vi "test_serialize_deserialize.vi"   [LabVIEW 2020, in "Waveform(DBL) Array.lvlib"]
doc: "Version 0.1"
uses:
  <vilib>/ADAS Record/CustomDataTypes/Waveform(DBL) Array/Waveform(DBL) Array.lvlib
  <vilib>/addons/_JKI Toolkits/Caraya/classes/Test/Test.lvclass
  <vilib>/addons/_JKI Toolkits/Caraya/classes/Assert/Assert.lvclass
  <vilib>/ADAS Record/CustomDataTypes/Waveform(DBL) Array/Process Data.ctl
  <vilib>/ADAS Record/CustomDataTypes/ADAS Generic/Serialize Data.vi
  <vilib>/ADAS Record/CustomDataTypes/ADAS Generic/NI_ADAS_Generic.lvlib
  <vilib>/ADAS Record/CustomDataTypes/ADAS Generic/Deserialize Data.vi
types:
  T1 = typedef "Waveform(DBL) Array.lvlib/Process Data.ctl" = cluster{"Waveform(dbl) Array":waveform(dbl)[]}
  T2 = typedef "NI_ADAS_Generic.lvlib/Process Data.ctl" = cluster{"Timestamp":timestamp, "Bus Channel":u16, "Byte Array":u8[]}
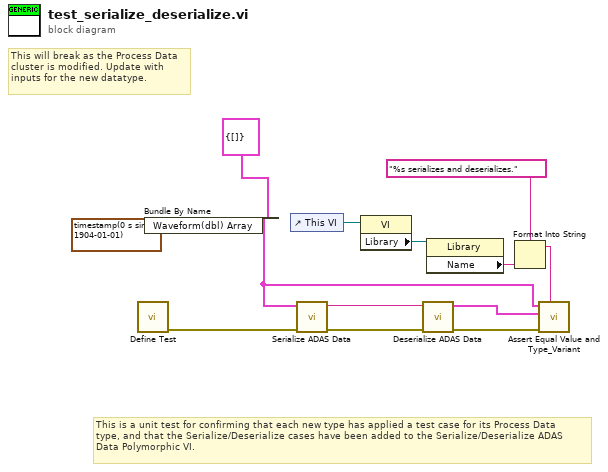
[diagram p0: block diagram]
diagram:
  # "This will break as the Process Data\ncluster is modified. Update with\ninputs for the new datatype."
  # "This is a unit test for confirming that each new type has applied a test case for its Process Data\ntype, and that the Serialize/Deserialize cases have been added to the Serialize/Deserialize ADAS\nData Polymorphic VI."
  n1 = call <vilib>:"Define Test.vi"() -> ("error out"=w8:errorcluster)  [unwired: 11 in]
  n2 = Bundle By Name "Bundle By Name"(cluster=T1 {"Waveform(dbl) Array"=[]} ("Process Data in"), "Waveform(dbl) Array"=timestamp(0 s since 1904-01-01) ("Timestamp")) -> (w2:T1)
  n3 = control-ref of="This VI"() -> (w13:refnum<vi>)
  n4 = call-poly <vilib>:"Serialize ADAS Data.vi"("error in (no error)"=w8, "Process Data"=w2) -> ("error out"=w7:errorcluster, "Flat Data out"=w6:string)  [unwired: 8 in]
  n5 = property class="VI"(reference=w13) -> ("Library"=w12:refnum<vi>)  [unwired: 1 in, 2 out]
  n6 = call-poly <vilib>:"Deserialize ADAS Data.vi"("error in (no error)"=w7, "Flat Data in"=w6) -> ("error out"=w4:errorcluster, "Process Data out"=w5:T2)  [unwired: 8 in]
  n7 = property class="Library"(reference=w12) -> ("Name"=w10:string)  [unwired: 1 in, 2 out]
  n8 = Format Into String(format string="%s serializes and deserializes.", w10) -> (resulting string=w9:string)  [unwired: 2 in, 1 out]
  n9 = call <vilib>:"Assert Equal Value and Type_Variant.vi"("Label"=w9, "error in (no error)"=w4, "Y"=w5, "X"=w2) -> ()  [unwired: 7 in, 1 out]
